vi "McP789A-SimpleMove-v0.80.vi"(0 "New Counter Position":dbl=10000.0 min=0.0 max=26000.0 format="%.2f", 11 "error in (no error)":errorcluster, 13 "Grating factor":dbl=10.0 min=0.1 max=100.0 format="%.2f") -> (4 "Final CounterRdg":dbl=10000.0 min=0.0 max=26000.0 format="%.2f", 8 "Final Wavelenth(nm)":dbl=1000.0 format="%.2f", 10 "Final Stepper Position":i32=-1000000, 15 "error out":errorcluster)   [LabVIEW 2019]
doc: "McP 789A-3 mover. Needs new counter position and velocity input, it reads current counter position from disk and save the final position back to disk."
uses:
  Globals and TypeDefs/Global Varibal Control.vi
panel:
  out "Current stepPos":i32=-1125000
  out "New Wavelength(nm)":dbl=1000.0 min=0.0 max=100000.0 format="%.3f"
  out "DelayTime":dbl=10.0 format="%.3f"
  out "Current CounterRdg":dbl=9500.0 min=0.0 max=26000.0 format="%.3f"
  out "Current Wavelength(nm)":dbl=950.0 min=0.0 max=100000.0 format="%.3f"
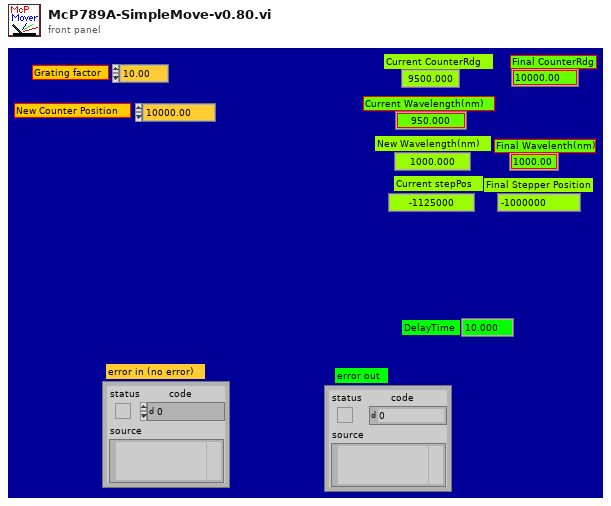
[diagram p1: front panel]
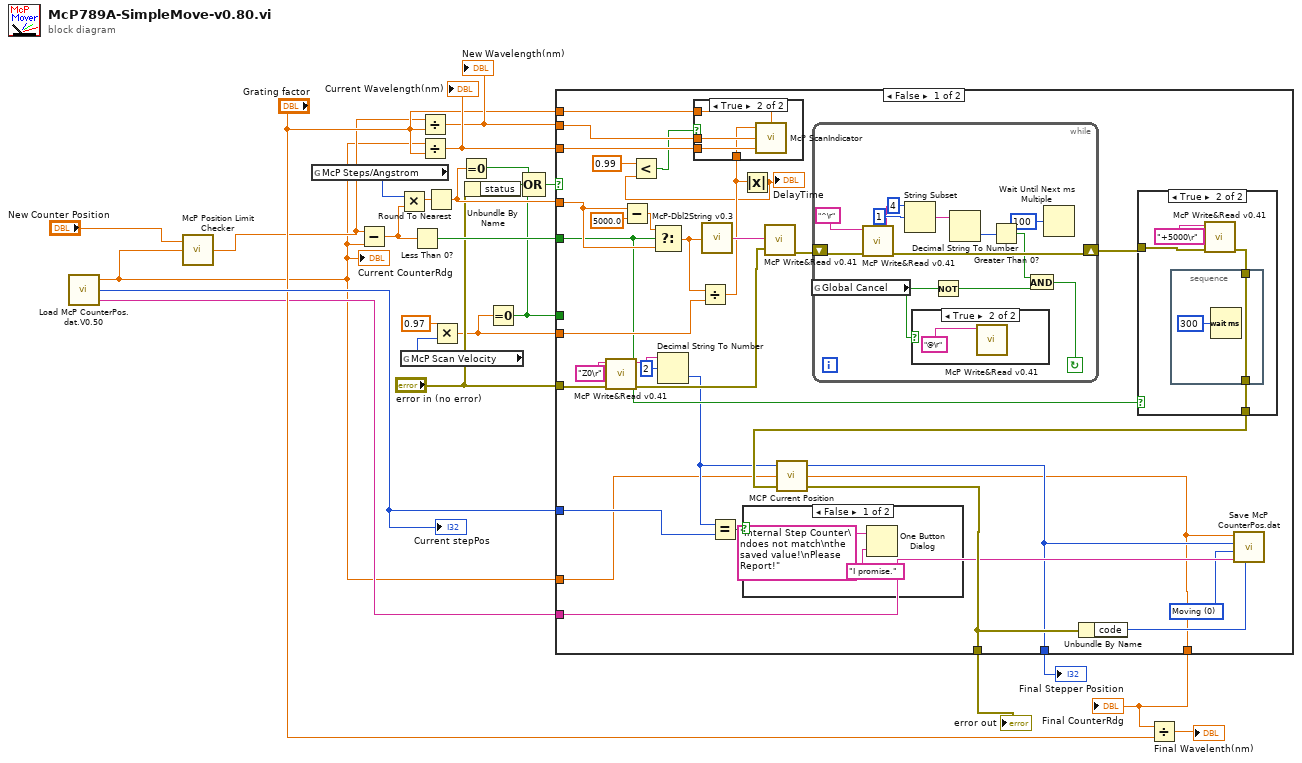
[diagram p0: block diagram]
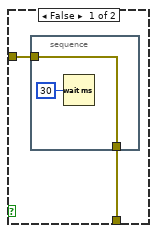
[diagram p5: hidden frame]
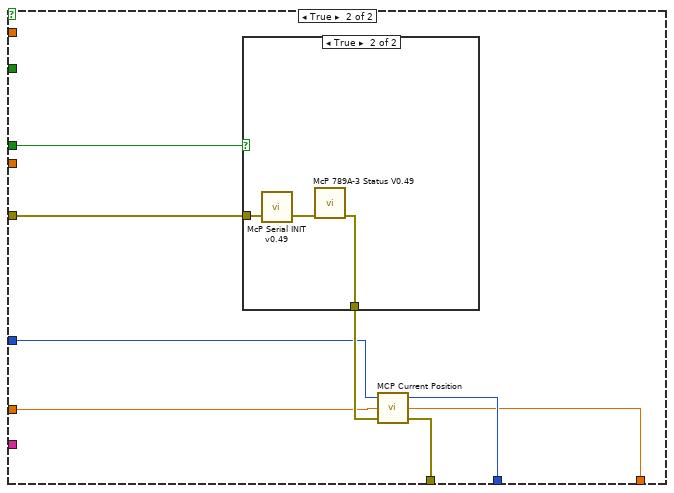
[diagram p6: hidden frame]
diagram:
  n1 = call "Load McP CounterPos.dat.V0.50.vi"() -> ("Counter Position"=w1:dbl, "Stepper Position"=w22:i32, "Last Calibration Date"=w8:string)  [unwired: 1 in]
  "Current CounterRdg" <- w1
  "Current stepPos" <- w22
  n2 = call "McP Position Limit Checker.vi"("Old Counter Position"=w1, "New Counter Position"="New Counter Position") -> ("New Counter Position output"=w3:dbl)  [unwired: 1 in]
  n3 = global read "Global Varibal Control.vi" "McP Steps/Angstrom"() -> (w5:i32)
  n4 = Subtract(x=w3, y=w1) -> (x-y=w23:dbl)
  n5 = Multiply(x=w5, y=w23) -> (x*y=w18:dbl)
  n6 = global read "Global Varibal Control.vi" "McP Scan Velocity"() -> (w4:i32)
  n7 = Less Than 0?(x=w23) -> (x < 0?=w24:bool)
  n8 = Divide(x=w3, y="Grating factor") -> (x/y=w20:dbl)
  "New Wavelength(nm)" <- w20
  n9 = Divide(x=w1, y="Grating factor") -> (x/y=w21:dbl)
  "Current Wavelength(nm)" <- w21
  n10 = Round To Nearest(number=w18) -> (nearest integer value=w17:dbl)
  n11 = Multiply(x=0.97, y=w4) -> (x*y=w7:dbl)
  n12 = Equal To 0?(x=w17) -> (x = 0?=w13:bool)
  n13 = Unbundle By Name("error in (no error)") -> ("status"=w14:bool)
  n14 = Equal To 0?(x=w7) -> (x = 0?=w6:bool)
  n15 = Compound Arithmetic op=OR(w13, w14, w6) -> (w12:bool)
  n16 = case shown="False" w12 {
    tunnel: w24 -> [w51 _]
    tunnel: w17 -> [w56 _]
    tunnel: w7 -> [w52 _]
    tunnel: "Grating factor" -> [w43 _]
    tunnel: w20 -> [w41 _]
    tunnel: w21 -> [w42 _]
    tunnel: w22 -> [w45 w91]
    tunnel: w1 -> [w35 w92]
    tunnel: [w26 w89] -> w10
    tunnel: "error in (no error)" -> [w47 w94]
    tunnel: [w27 w90] -> w9
    tunnel: [w37 w88] -> w16
    tunnel: w8 -> [w29 _]
    tunnel: w6 -> [_ w95]
    frame False {
      w28 = u16 0 items=["Moving", "Calibration", "Key in", "Initialization"] ("Set Method")
      n17 = call "McP Write&Read v0.41.vi"("error in (no error)"=w47, "Write String"="Z0\r") -> ("error out"=w46:errorcluster, "Read String\nshows:"=w49:string)  [unwired: 2 in, 3 out]
      n18 = Subtract(x=w56, y=5000.0) -> (x-y=w55:dbl)
      n19 = Select(t=w55, s=w51, f=w56) -> (s? t:f=w53:dbl)
      n20 = Decimal String To Number(string=w49, offset=2) -> (number=w36:i32)  [unwired: 1 in, 1 out]
      n21 = Divide(x=w53, y=w52) -> (x/y=w32:dbl)
      n22 = call "McP-Dbl2String v0.3.vi"("McP Input Number"=w53) -> ("Controller String"=w54:string)
      n23 = Equal?(x=w36, y=w45) -> (x = y?=w44:bool)
      n24 = Absolute Value(x=w32) -> (abs(x)=w31:dbl)
      "DelayTime" <- w31
      n25 = Less?(x=0.99, y=w31) -> (x < y?=w33:bool)
      n26 = case shown="True" w33 {
        tunnel: w43 -> [_ w75]
        tunnel: w42 -> [_ w74]
        tunnel: w41 -> [_ w73]
        tunnel: w32 -> [_ w72]
        frame False {
        }
        frame True {
          n27 = call "McP ScanIndicator.vi"("Grating factor"=w75, "Current Wavelength"=w74, "New Wavelength"=w73, "MoveTime(ms)"=w72) -> ()  [unwired: 1 in]
        }
      }
      n28 = case shown="False" w44 {
        frame False {
          n29 = One Button Dialog(message="Internal Step Counter\ndoes not match\nthe saved value!\nPlease Report!", button name ("OK")="I promise.") -> ()  [unwired: 1 out]
        }
        frame True {
        }
      }
      n30 = call "McP Write&Read v0.41.vi"("error in (no error)"=w46, "Write String"=w54) -> ("error out"=w40:errorcluster)  [unwired: 2 in, 4 out]
      n31 = while {
        shift-left: w40 -> [w70]
        shift-right: [w69] -> w39
        stop <- w61 continue-if-true
        n32 = global read "Global Varibal Control.vi" "Global Cancel"() -> (w58:bool)
        n33 = call "McP Write&Read v0.41.vi"("error in (no error)"=w70, "Write String"="^\r") -> ("error out"=w69:errorcluster, "Read String\nshows:"=w65:string)  [unwired: 2 in, 3 out]
        n34 = String Subset(string=w65, offset (0)=1, length (rest)=4) -> (substring=w64:string)
        n35 = case shown="True" w58 {
          frame False {
          }
          frame True {
            n36 = call "McP Write&Read v0.41.vi"("Write String"="@\r") -> ()  [unwired: 3 in, 5 out]
          }
        }
        n37 = Not(x=w58) -> (.not. x?=w59:bool)
        n38 = Decimal String To Number(string=w64) -> (number=w62:i32)  [unwired: 2 in, 1 out]
        n39 = Greater Than 0?(x=w62) -> (x > 0?=w60:bool)
        n40 = And(x=w60, y=w59) -> (x .and. y?=w61:bool)
        n41 = Wait Until Next ms Multiple(millisecond multiple=u32 100) -> ()  [unwired: 1 out]
      }
      n42 = case shown="True" w51 {
        tunnel: w39 -> [w79 w84]
        tunnel: [w78 w82] -> w38
        frame False {
          n43 = stacked-sequence {
            tunnel: [w80] -> w78
            tunnel: w79 -> [w80]
            frame #0 {
              n44 = Wait (ms)(milliseconds to wait=u32 30) -> ()  [unwired: 1 out]
            }
          }
        }
        frame True {
          n45 = call "McP Write&Read v0.41.vi"("error in (no error)"=w84, "Write String"="+5000\r") -> ("error out"=w83:errorcluster)  [unwired: 2 in, 4 out]
          n46 = stacked-sequence {
            tunnel: w83 -> [w86]
            tunnel: [w86] -> w82
            frame #0 {
              n47 = Wait (ms)(milliseconds to wait=u32 300) -> ()  [unwired: 1 out]
            }
          }
        }
      }
      n48 = call "MCP Current Position.vi"("error in (no error)"=w38, "Initial Couter Reading"=w35, "Initial Stepper Position"=w36) -> ("error out"=w37:errorcluster, "Current Couter Reading"=w26:dbl, "Current Stepper Position"=w27:i32)
      n49 = Unbundle By Name(w37) -> ("code"=w30:i32)
      n50 = call "Save McP CounterPos.dat.vi"("Error Code (0: No Error)"=w30, "Last Calibration Date"=w29, "Set Method"=w28, "McP Stepper Position"=w27, "McP Counter Position"=w26) -> ()  [unwired: 1 in, 1 out]
    }
    frame True {
      n51 = case shown="True" w95 {
        tunnel: w94 -> [w96 w98]
        tunnel: [w96 w97] -> w93
        frame False {
        }
        frame True {
          n52 = call "McP Serial INIT v0.49.vi"("error in (no error)"=w98) -> ("Error out"=w99:errorcluster)  [unwired: 1 in, 1 out]
          n53 = call "McP 789A-3 Status V0.49.vi"("error in (no error)"=w99) -> ("error out"=w97:errorcluster)  [unwired: 7 in, 3 out]
        }
      }
      n54 = call "MCP Current Position.vi"("error in (no error)"=w93, "Initial Couter Reading"=w92, "Initial Stepper Position"=w91) -> ("error out"=w88:errorcluster, "Current Couter Reading"=w89:dbl, "Current Stepper Position"=w90:i32)
    }
  }
  "Final CounterRdg" <- w10
  "Final Stepper Position" <- w9
  "error out" <- w16
  n55 = Divide(x=w10, y="Grating factor") -> (x/y=→"Final Wavelenth(nm)":dbl)
